vi "Actor Core.vi"(8 "error in":errorcluster, 11 "RFSA DAQ in":refnum<class "RFSA DAQ.lvclass">) -> (0 "error out":errorcluster, 3 "Actor out":refnum<class "Actor.lvclass">)   [LabVIEW 2025, in "RFSA DAQ.lvlib" / "RFSA DAQ.lvclass"]
doc: "<p>(<strong>Filename</strong>: <span class=\"dnl\">Actor Framework.lvlib:Actor.lvclass:Actor Core.vi</span>)</p>\n<p>Receives messages to the actor, reacts to them, and initiates any error handling that may shut the actor down.</p>\n<p>Descendant classes may override this VI to append parallel tasks for the actor to complete while it handles messages. Overrides use the <a href=\"nihelplauncher://docs/csh?context=lvcore_glang_udclass\">Call Parent Class Method</a> node.</p>"
uses:
  RFSA DAQ.lvclass
  RFSA DAQ.lvclass/RFSA DAQ.ctl
  DAQ Interface/DAQ Interface/DAQ Interface.lvclass
  Helper Loop Type.ctl
  Helper Loop Message.ctl
  <vilib>/ActorFramework/Actor/Actor.lvclass
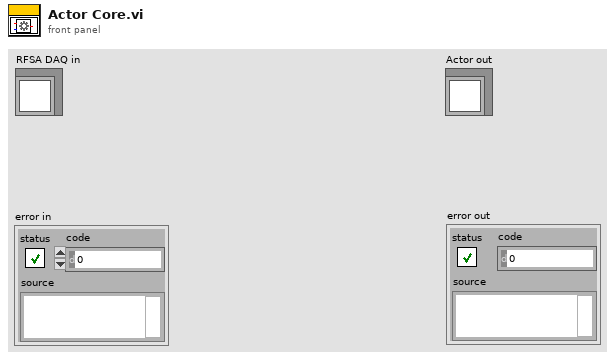
[diagram p1: front panel]
types:
  T1 = typedef "RFSA DAQ.lvlib/RFSA DAQ.lvclass/Helper Loop Message.ctl" = cluster{"Type":T2, "Payload":variant}
  T2 = typedef "RFSA DAQ.lvlib/RFSA DAQ.lvclass/Helper Loop Type.ctl" = enum16{"Configure", "Start", "Do", "Stop", "Clean", "Close"}
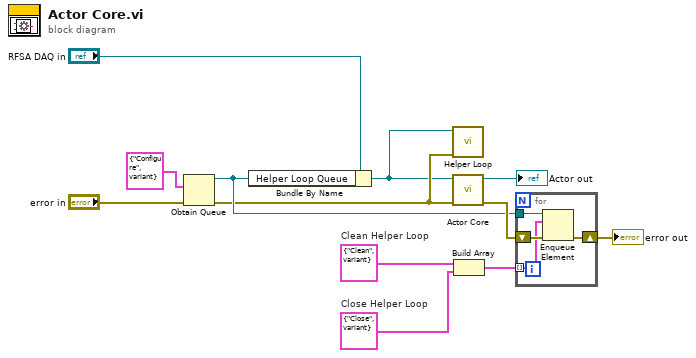
[diagram p0: block diagram]
diagram:
  w3 = T1 {"Type"=enum."Close", "Payload"=variant}  # Close Helper Loop
  w4 = T1 {"Type"=enum."Clean", "Payload"=variant}  # Clean Helper Loop
  n1 = Obtain Queue(element data type=T1 {"Type"=enum."Configure", "Payload"=variant} ("Message"), error in (no error)="error in") -> (queue out=w5:refnum<queue>, error out=w2:errorcluster)  [unwired: 3 in, 1 out]
  n2 = Bundle By Name(cluster="RFSA DAQ in", "Helper Loop Queue"=w5) -> (w1:refnum<class "RFSA DAQ.lvclass">)
  n3 = call "Helper Loop.vi"("error in (no error)"=w2, "RFSA DAQ in"=w1) -> ()  [unwired: 10 in]
  n4 = call-parent "Actor Core.vi"("error in"=w2, "Actor in"=w1) -> ("error out"=w12:errorcluster, "Actor out"=→"Actor out":refnum<class "Actor.lvclass">)  [unwired: 8 in]
  n5 = Build Array(w4, w3) -> (w11:T1[])
  n6 = for {
    tunnel: w5 -> [w15]
    tunnel: w11 -> [w13] mode=indexing
    shift-right: [w14] -> w10
    shift-left: w12 -> [w16]
    n7 = Enqueue Element(queue=w15, element=w13, error in (no error)=w16) -> (error out=w14:errorcluster)  [unwired: 1 in, 2 out]
  }
  "error out" <- w10
